vi "ep_Check Error (1 CH).vi"(8 "error in (no error)":errorcluster, 9 "fundamental frequency [Hz]":dbl=50.0, 10 "slip":dbl, 11 "spectra":T1) -> (0 "error out":errorcluster, 1 "dup fundamental frequency [Hz]":dbl=50.0, 2 "dup slip":dbl, 3 "dup spectra":T1, 4 "valid for detection?":bool)   [LabVIEW 2014, in "NI_EP_Motor Monitoring.lvlib"]
uses:
  <vilib>/addons/Electrical Power/Motor Monitoring/NI_EP_Motor Monitoring.lvlib
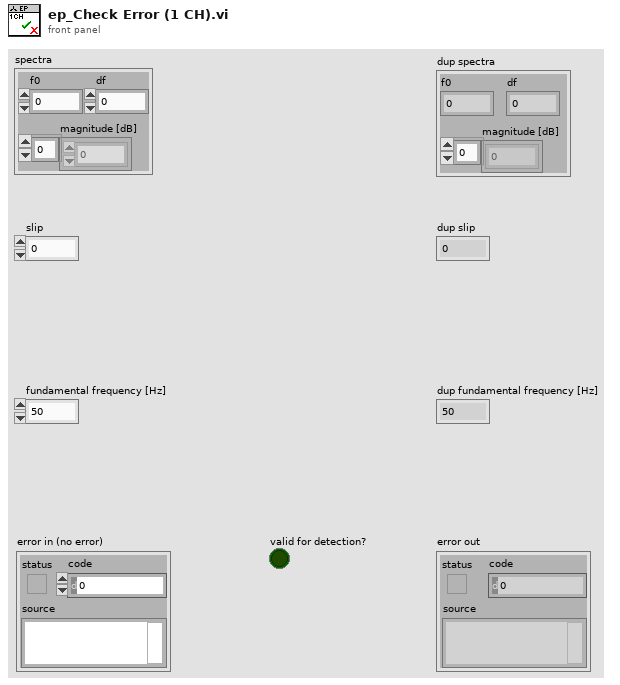
[diagram p1: front panel]
types:
  T1 = cluster{"f0":dbl, "df":dbl, "magnitude [dB]":dbl[]}
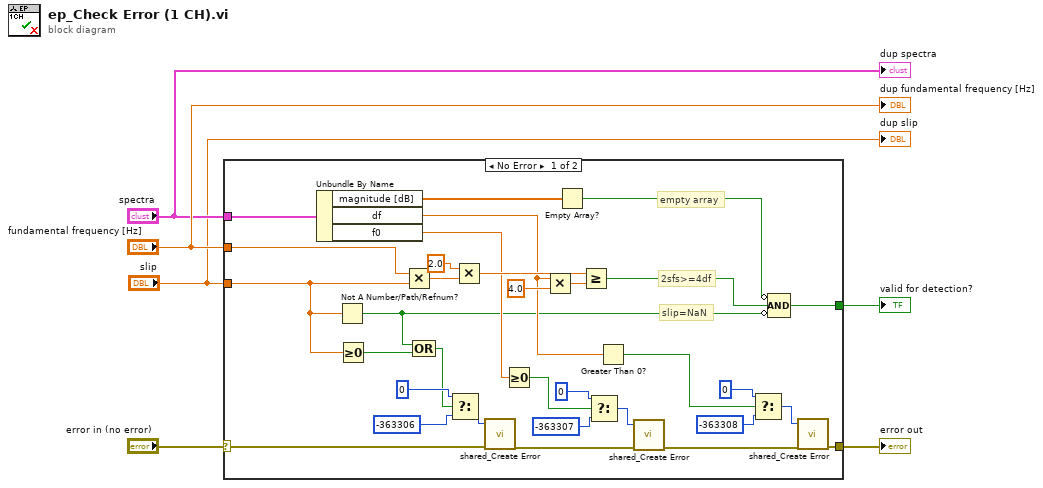
[diagram p0: block diagram]
diagram:
  n1 = case shown="No Error" "error in (no error)" {
    selector: "error in (no error)" -> [w29 w39]
    tunnel: "spectra" -> [w33 _]
    tunnel: [w23 w39] -> w4
    tunnel: "slip" -> [w9 _]
    tunnel: "fundamental frequency [Hz]" -> [w10 _]
    tunnel: [w12 _] -> w5
    frame No Error {
      # "empty array"
      # "2sfs>=4df"
      # "slip=NaN"
      n2 = Unbundle By Name(w33) -> ("magnitude [dB]"=w8:dbl[], "df"=w28:dbl, "f0"=w17:dbl)
      n3 = Not A Number/Path/Refnum?(number/path/refnum=w9) -> (NaN/Path/Refnum?=w14:bool)
      n4 = Greater Or Equal To 0?(x=w9) -> (x >= 0?=w11:bool)
      n5 = Multiply(x=w10, y=w9) -> (x*y=w38:dbl)
      n6 = Compound Arithmetic op=OR(w14, w11) -> (w15:bool)
      n7 = Select(t=0 ("error code (0)"), s=w15, f=-363306 ("error code (0)")) -> (s? t:f=w31:i32)
      n8 = Multiply(x=2.0, y=w38) -> (x*y=w35:dbl)
      n9 = call <vilib>:"shared_Create Error.vi"("error in (no error)"=w29, "error code (0)"=w31) -> ("error out"=w19:errorcluster)  [unwired: 9 in]
      n10 = Greater Or Equal To 0?(x=w17) -> (x >= 0?=w16:bool)
      n11 = Multiply(x=w28, y=4.0) -> (x*y=w34:dbl)
      n12 = Empty Array?(array=w8) -> (empty?=w7:bool)
      n13 = Greater Or Equal?(x=w35, y=w34) -> (x >= y?=w13:bool)
      n14 = Select(t=0 ("error code (0)"), s=w16, f=-363307 ("error code (0)")) -> (s? t:f=w21:i32)
      n15 = Greater Than 0?(x=w28) -> (x > 0?=w24:bool)
      n16 = call <vilib>:"shared_Create Error.vi"("error in (no error)"=w19, "error code (0)"=w21) -> ("error out"=w18:errorcluster)  [unwired: 9 in]
      n17 = Select(t=0 ("error code (0)"), s=w24, f=-363308 ("error code (0)")) -> (s? t:f=w26:i32)
      n18 = Compound Arithmetic op=AND(invert w7, w13, invert w14) -> (w12:bool)
      n19 = call <vilib>:"shared_Create Error.vi"("error in (no error)"=w18, "error code (0)"=w26) -> ("error out"=w23:errorcluster)  [unwired: 9 in]
    }
    frame Error {
    }
  }
  "error out" <- w4
  "valid for detection?" <- w5
  "dup spectra" <- "spectra"
  "dup fundamental frequency [Hz]" <- "fundamental frequency [Hz]"
  "dup slip" <- "slip"
